vi "XH转换.vi"(11 "XH":string="34040000001020012018103012") -> (3 "xh输出":string)   [LabVIEW 2016]
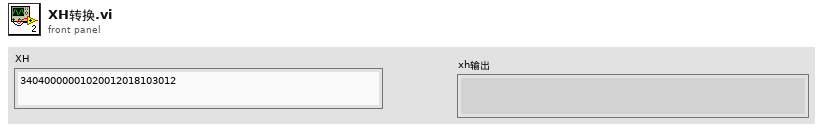
[diagram p1: front panel]
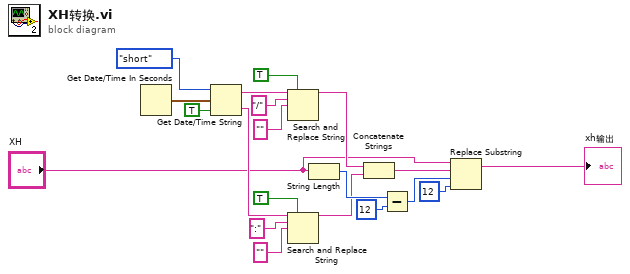
[diagram p0: block diagram]
diagram:
  n1 = Get Date/Time In Seconds() -> (seconds since 1Jan1904=w18:timestamp)
  n2 = Get Date/Time String(date format (0)=enum16{"short", "long", "abbreviated"}."short" ("日期格式(0)"), seconds (now)=w18, want seconds? (F)=TRUE ("需要秒？(F)")) -> (date string=w17:string, time string=w10:string)
  n3 = Search and Replace String(replace all?=TRUE ("替换全部？(F)"), input string=w17, search string="/" ("搜索字符串"), replace string="" ("替换字符串(\"\")")) -> (result string=w7:string)  [unwired: 4 in, 3 out]
  n4 = Search and Replace String(replace all?=TRUE ("替换全部？(F)"), input string=w10, search string=":" ("搜索字符串"), replace string="" ("替换字符串(\"\")")) -> (result string=w6:string)  [unwired: 4 in, 3 out]
  n5 = String Length(string="XH") -> (length=w20:i32)
  n6 = Concatenate Strings(w7, w6) -> (w5:string)
  n7 = Subtract(x=w20, y=12) -> (x-y=w4:i32)
  n8 = Replace Substring(2:12 ("长度（子字符串长度）"), 3:w4, 4:w5, 5:"XH") -> (1:→"xh输出":string)  [unwired: 1 out]
